vi "NT Prepare Table Name.vi"(10 "Name":string, 11 "Table Prefix":string) -> (3 "Prefixed Name":string)   [LabVIEW 2025]
doc: "Construct the full variable name. Ensure / present on front and back of prefix and append name."
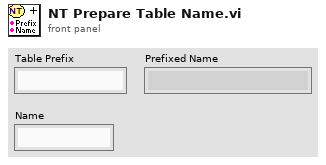
[diagram p1: front panel]
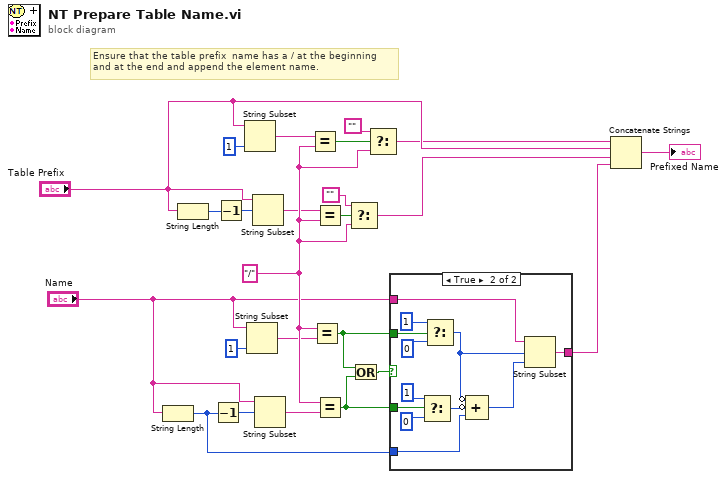
[diagram p0: block diagram]
diagram:
  w24 = "/"
  # "Ensure that the table prefix  name has a / at the beginning\nand at the end and append the element name."
  n1 = String Length(string="Name") -> (length=w6:i32)
  n2 = String Length(string="Table Prefix") -> (length=w17:i32)
  n3 = Decrement(x=w6) -> (x-1=w7:i32)
  n4 = Decrement(x=w17) -> (x-1=w18:i32)
  n5 = String Subset(string="Table Prefix", length (rest)=1 ("length (rest)")) -> (substring=w21:string)  [unwired: 1 in]
  n6 = String Subset(string="Name", length (rest)=1 ("length (rest)")) -> (substring=w12:string)  [unwired: 1 in]
  n7 = String Subset(string="Table Prefix", offset (0)=w18) -> (substring=w14:string)  [unwired: 1 in]
  n8 = String Subset(string="Name", offset (0)=w7) -> (substring=w11:string)  [unwired: 1 in]
  n9 = Equal?(x=w21, y=w24) -> (x = y?=w20:bool)
  n10 = Equal?(x=w24, y=w12) -> (x = y?=w9:bool)
  n11 = Equal?(x=w14, y=w24) -> (x = y?=w16:bool)
  n12 = Equal?(x=w24, y=w11) -> (x = y?=w8:bool)
  n13 = Select(t="", s=w16, f=w24) -> (s? t:f=w2:string)
  n14 = Or(x=w9, y=w8) -> (x .or. y?=w10:bool)
  n15 = Select(t="", s=w20, f=w24) -> (s? t:f=w1:string)
  n16 = case shown="True" w10 {
    tunnel: "Name" -> [w25 w36]
    tunnel: [w25 w37] -> w23
    tunnel: w9 -> [_ w35]
    tunnel: w8 -> [_ w32]
    tunnel: w6 -> [_ w27]
    frame False {
    }
    frame True {
      n17 = Select(t=1 ("length (rest)"), s=w32, f=0 ("length (rest)")) -> (s? t:f=w29:i32)
      n18 = Select(t=1 ("length (rest)"), s=w35, f=0 ("length (rest)")) -> (s? t:f=w28:i32)
      n19 = Compound Arithmetic op=ADD(invert w28, invert w29, w27) -> (w26:i32)
      n20 = String Subset(string=w36, offset (0)=w28, length (rest)=w26) -> (substring=w37:string)
    }
  }
  n21 = Concatenate Strings(w1, "Table Prefix", w2, w23) -> (→"Prefixed Name":string)
